vi "plot_close.vi"(11 "Close?":bool) -> ()   [LabVIEW 2019]
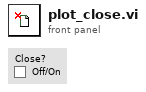
[diagram p1: front panel]
types:
  T1 = enum32{"Invalid", "Standard", "Closed", "Hidden", "Minimized", "Maximized"}
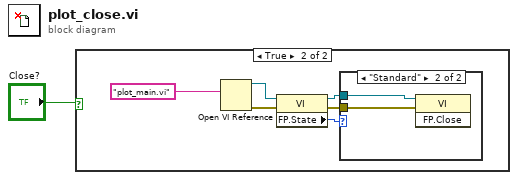
[diagram p0: block diagram]
diagram:
  n1 = case shown="True" "Close?" {
    frame False {
    }
    frame True {
      n2 = Open VI Reference(vi path="plot_main.vi") -> (vi reference=w6:refnum<vi>, error out=w7:errorcluster)  [unwired: 5 in]
      n3 = property class="VI"(reference=w6, error in=w7) -> (reference out=w4:refnum<vi>, error out=w5:errorcluster, "FP.State"=w3:T1)
      n4 = case shown="\"Standard\"" w3 {
        tunnel: w4 -> [_ w9]
        tunnel: w5 -> [_ w8]
        frame "Invalid", Default {
        }
        frame "Standard" {
          n5 = invoke class="VI" method="FP.Close"(reference=w9, error in=w8) -> ()  [unwired: 1 in, 3 out]
        }
      }
    }
  }
